vi "ParseData.vi"(9 "data out":string) -> (0 "Sensor data 5":cluster{"sp float":u16, "sp float":u16}, 1 "Sensor data 3":cluster{"sp float":u16, "sp float":u16}, 2 "Sensor data 2":cluster{"sp float":u16, "sp float":u16}, 3 "Sensor data 1":cluster{"sp float":u16, "sp float":u16}, 4 "Sensor data 4":cluster{"sp float":u16, "sp float":u16}, 5 "Sensor data 6":cluster{"sp float":u16, "sp float":u16}, 8 "Sensor Id":T2, 11 "GTS Fields":T1)   [LabVIEW 2011]
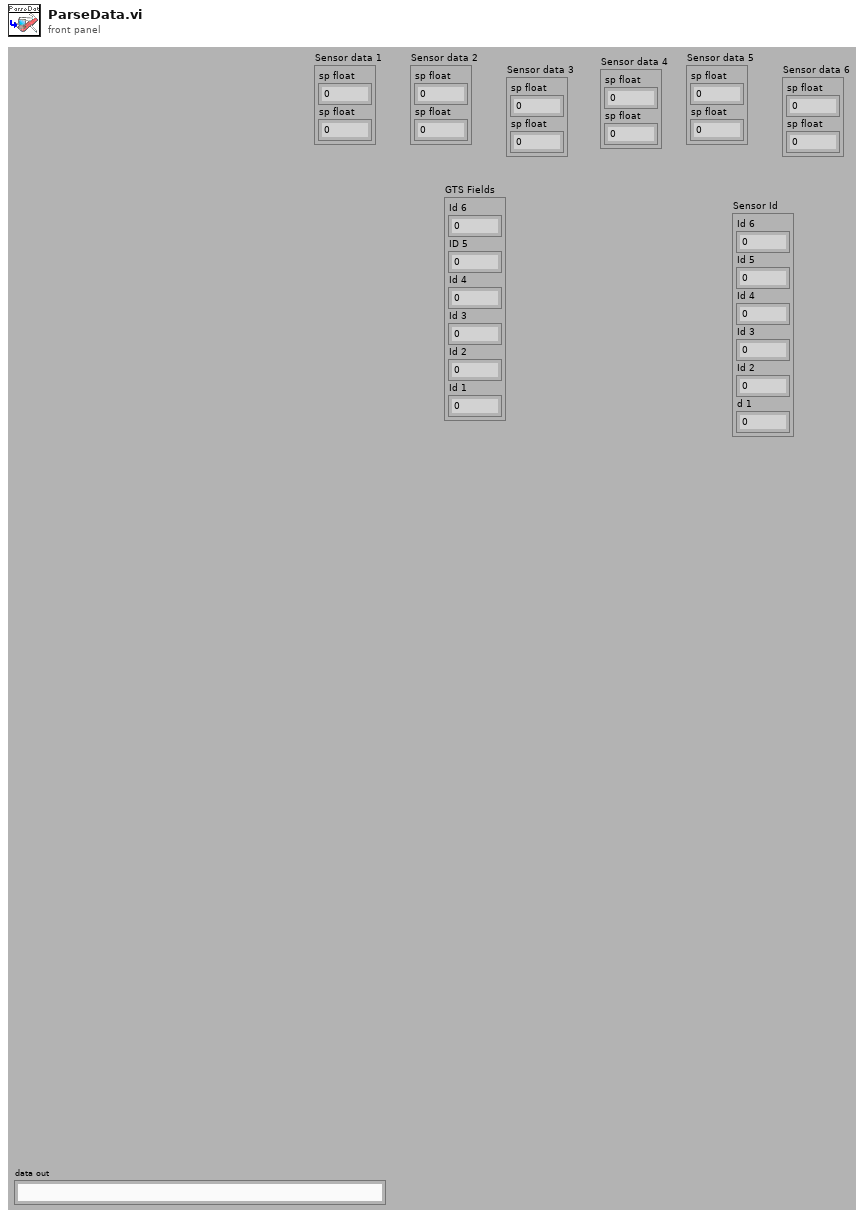
[diagram p1: front panel]
types:
  T1 = cluster{"Id 6":u8, "ID 5":u8, "Id 4":u8, "Id 3":u8, "Id 2":u8, "Id 1":u8}
  T2 = cluster{"Id 6":u8, "Id 5":u8, "Id 4":u8, "Id 3":u8, "Id 2":u8, "d 1":u8}
  T3 = cluster{"sp float":u8, "sp float":u8, "sp float":u8, "sp float":u8, "sp float":u8, "sp float":u8}
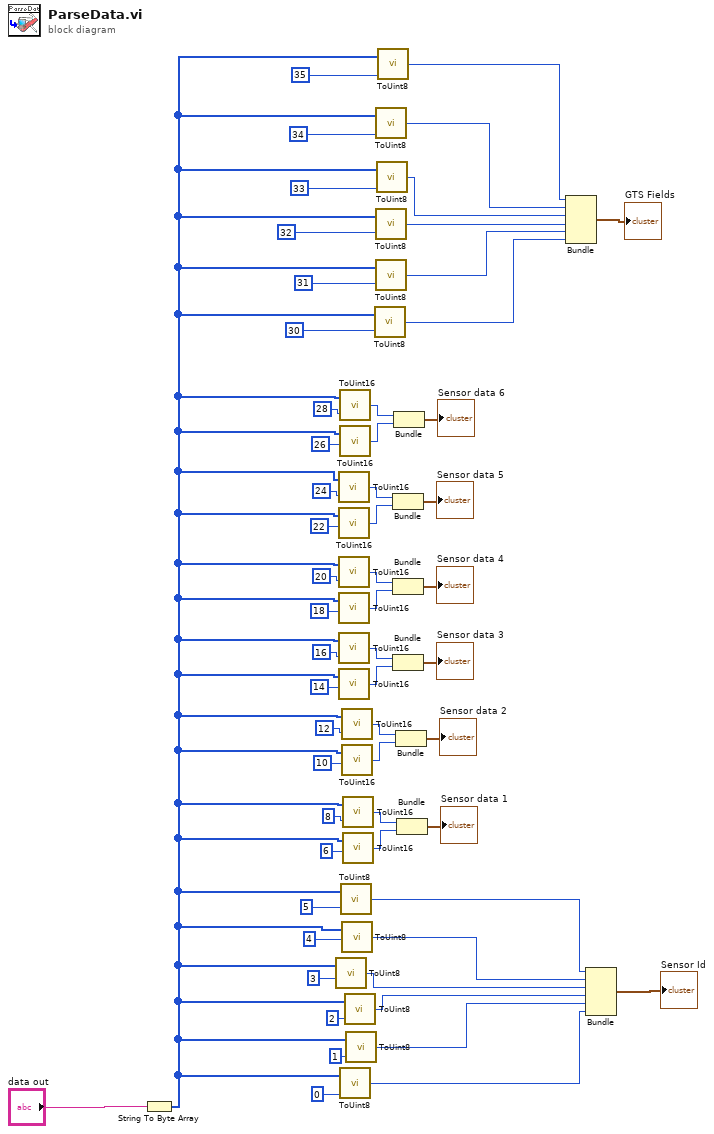
[diagram p0: block diagram]
diagram:
  n1 = String To Byte Array(string="data out") -> (unsigned byte array=w1:u8[])
  n2 = call "ToUint8.vi"("index"=3, "array"=w1) -> ("sp float"=w41:u8)
  n3 = call "ToUint16.vi"("index"=24, "array"=w1) -> ("sp float"=w9:u16)
  n4 = call "ToUint16.vi"("index"=22, "array"=w1) -> ("sp float"=w10:u16)
  n5 = call "ToUint16.vi"("index"=20, "array"=w1) -> ("sp float"=w23:u16)
  n6 = call "ToUint16.vi"("index"=18, "array"=w1) -> ("sp float"=w24:u16)
  n7 = call "ToUint16.vi"("index"=16, "array"=w1) -> ("sp float"=w28:u16)
  n8 = call "ToUint16.vi"("index"=14, "array"=w1) -> ("sp float"=w27:u16)
  n9 = call "ToUint16.vi"("index"=28, "array"=w1) -> ("sp float"=w4:u16)
  n10 = call "ToUint16.vi"("index"=26, "array"=w1) -> ("sp float"=w5:u16)
  n11 = call "ToUint8.vi"("index"=0, "array"=w1) -> ("sp float"=w38:u8)
  n12 = call "ToUint8.vi"("index"=5, "array"=w1) -> ("sp float"=w43:u8)
  n13 = call "ToUint16.vi"("index"=12, "array"=w1) -> ("sp float"=w33:u16)
  n14 = call "ToUint16.vi"("index"=10, "array"=w1) -> ("sp float"=w34:u16)
  n15 = call "ToUint8.vi"("index"=4, "array"=w1) -> ("sp float"=w42:u8)
  n16 = call "ToUint16.vi"("index"=8, "array"=w1) -> ("sp float"=w53:u16)
  n17 = call "ToUint16.vi"("index"=6, "array"=w1) -> ("sp float"=w52:u16)
  n18 = call "ToUint8.vi"("index"=2, "array"=w1) -> ("sp float"=w40:u8)
  n19 = call "ToUint8.vi"("index"=1, "array"=w1) -> ("sp float"=w39:u8)
  n20 = call "ToUint8.vi"("index"=30, "array"=w1) -> ("sp float"=w13:u8)
  n21 = call "ToUint8.vi"("index"=34, "array"=w1) -> ("sp float"=w17:u8)
  n22 = call "ToUint8.vi"("index"=32, "array"=w1) -> ("sp float"=w15:u8)
  n23 = call "ToUint8.vi"("index"=31, "array"=w1) -> ("sp float"=w14:u8)
  n24 = call "ToUint8.vi"("index"=33, "array"=w1) -> ("sp float"=w16:u8)
  n25 = call "ToUint8.vi"("index"=35, "array"=w1) -> ("sp float"=w18:u8)
  n26 = Bundle("sp float"=w9, "sp float"=w10) -> (→"Sensor data 5":cluster{"sp float":u16, "sp float":u16})  [unwired: 1 in]
  n27 = Bundle("sp float"=w23, "sp float"=w24) -> (→"Sensor data 4":cluster{"sp float":u16, "sp float":u16})  [unwired: 1 in]
  n28 = Bundle("sp float"=w28, "sp float"=w27) -> (→"Sensor data 3":cluster{"sp float":u16, "sp float":u16})  [unwired: 1 in]
  n29 = Bundle("sp float"=w4, "sp float"=w5) -> (→"Sensor data 6":cluster{"sp float":u16, "sp float":u16})  [unwired: 1 in]
  n30 = Bundle("sp float"=w33, "sp float"=w34) -> (→"Sensor data 2":cluster{"sp float":u16, "sp float":u16})  [unwired: 1 in]
  n31 = Bundle("sp float"=w53, "sp float"=w52) -> (→"Sensor data 1":cluster{"sp float":u16, "sp float":u16})  [unwired: 1 in]
  n32 = Bundle("sp float"=w18, "sp float"=w17, "sp float"=w16, "sp float"=w15, "sp float"=w14, "sp float"=w13) -> (→"GTS Fields":T3)  [unwired: 1 in]
  n33 = Bundle("sp float"=w43, "sp float"=w42, "sp float"=w41, "sp float"=w40, "sp float"=w39, "sp float"=w38) -> (→"Sensor Id":T3)  [unwired: 1 in]
